vi "7HP_Send Cmd, wait for ack.vi"(3 "Error In":errorcluster, 4 "Operation":T1="s", 5 "Port":refnum<visa-resource-name>) -> (0 "Error Out":errorcluster, 1 "ack ok":bool, 2 "Port out":refnum<visa-resource-name>)   [LabVIEW 2020]
uses:
  ctls/7HP_Cmd (USB).ctl
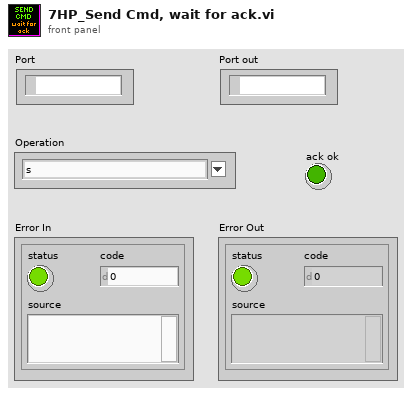
[diagram p1: front panel]
types:
  T1 = typedef "7HP_Cmd (USB).ctl" = string
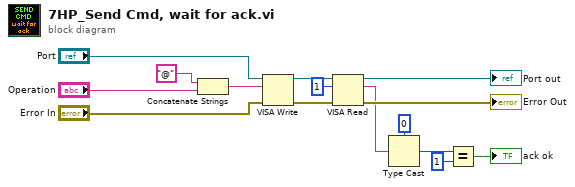
[diagram p0: block diagram]
diagram:
  n1 = Concatenate Strings("@", "Operation") -> (w14:string)
  n2 = VISA Write(VISA resource name="Port", write buffer=w14, error in (no error)="Error In") -> (VISA resource name out=w10:refnum<visa-resource-name>, error out=w9:errorcluster)  [unwired: 1 out]
  n3 = VISA Read(VISA resource name=w10, byte count=u32 1, error in (no error)=w9) -> (VISA resource name out=→"Port out":refnum<visa-resource-name>, read buffer=w5:string, error out=→"Error Out":errorcluster)  [unwired: 1 out]
  n4 = Type Cast(type=u8 0 ("byte count"), x=w5) -> (*(type *) &x=w3:u8)
  n5 = Equal?(x=w3, y=u8 1 ("byte count")) -> (x = y?=→"ack ok":bool)
